vi "ServerMessageParseStateMachine.vi"(0 "LastState":T3, 1 "LastDataBuffer":string, 2 "LastFrameState":T1, 5 "error in":errorcluster) -> (14 "CurrentState":T3, 15 "CurrentDataBuffer":string, 16 "CurrentFrameState":T1, 18 "ReadyFrames":T1[](array[typedef]), 19 "error out":errorcluster)   [LabVIEW 2017, in "STOMP.lvclass"]
uses:
  STOMP.lvclass
  Typedefs/Type_MessageParserState.ctl
  Typedefs/Type_ServerFrame.ctl
  Typedefs/Type_ServerFrameType.ctl
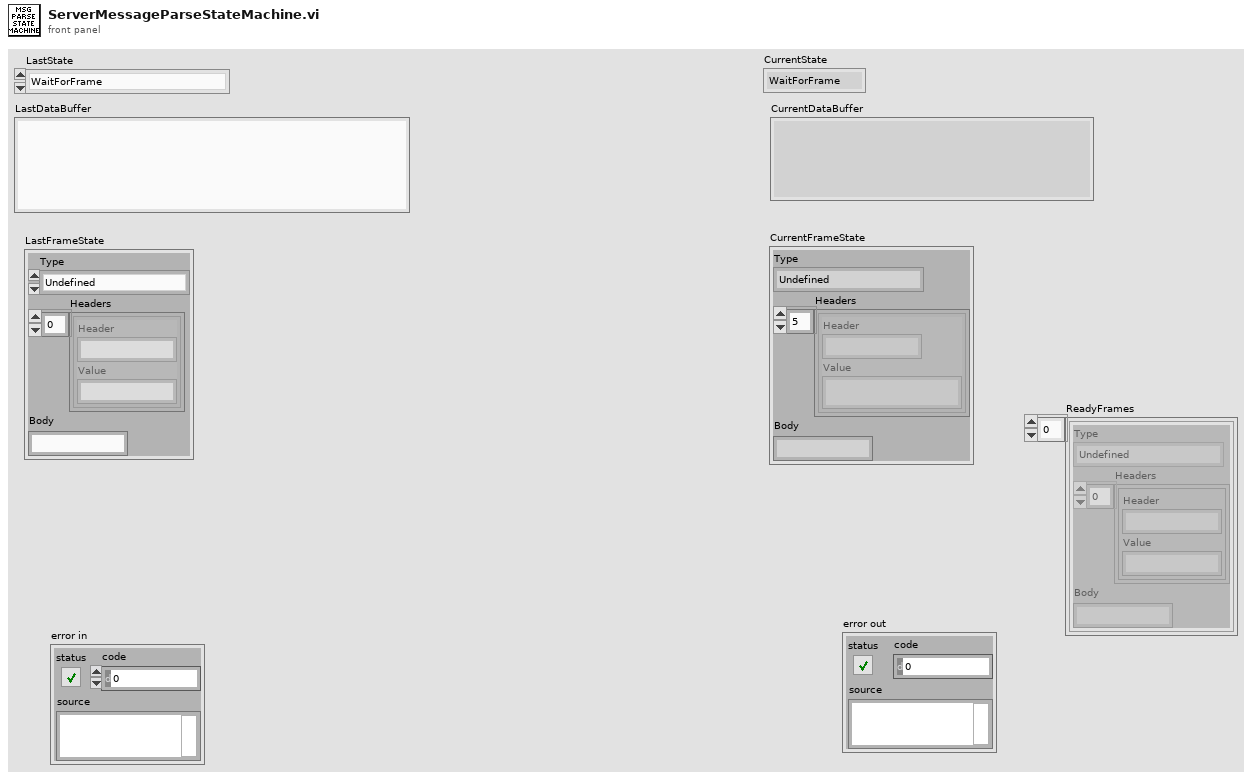
[diagram p1: front panel]
types:
  T1 = typedef "STOMP.lvclass/Type_ServerFrame.ctl" = cluster{"Type":T2, "Headers":cluster{"Header":string, "Value":string}[], "Body":string}
  T2 = typedef "STOMP.lvclass/Type_ServerFrameType.ctl" = enum16{"Undefined", "MESSAGE", "CONNECTED", "RECEIPT", "ERROR"}
  T3 = typedef "STOMP.lvclass/Type_MessageParserState.ctl" = enum16{"WaitForFrame", "ReadCommand", "ReadHeaders", "ReadBody", "FrameReady"}
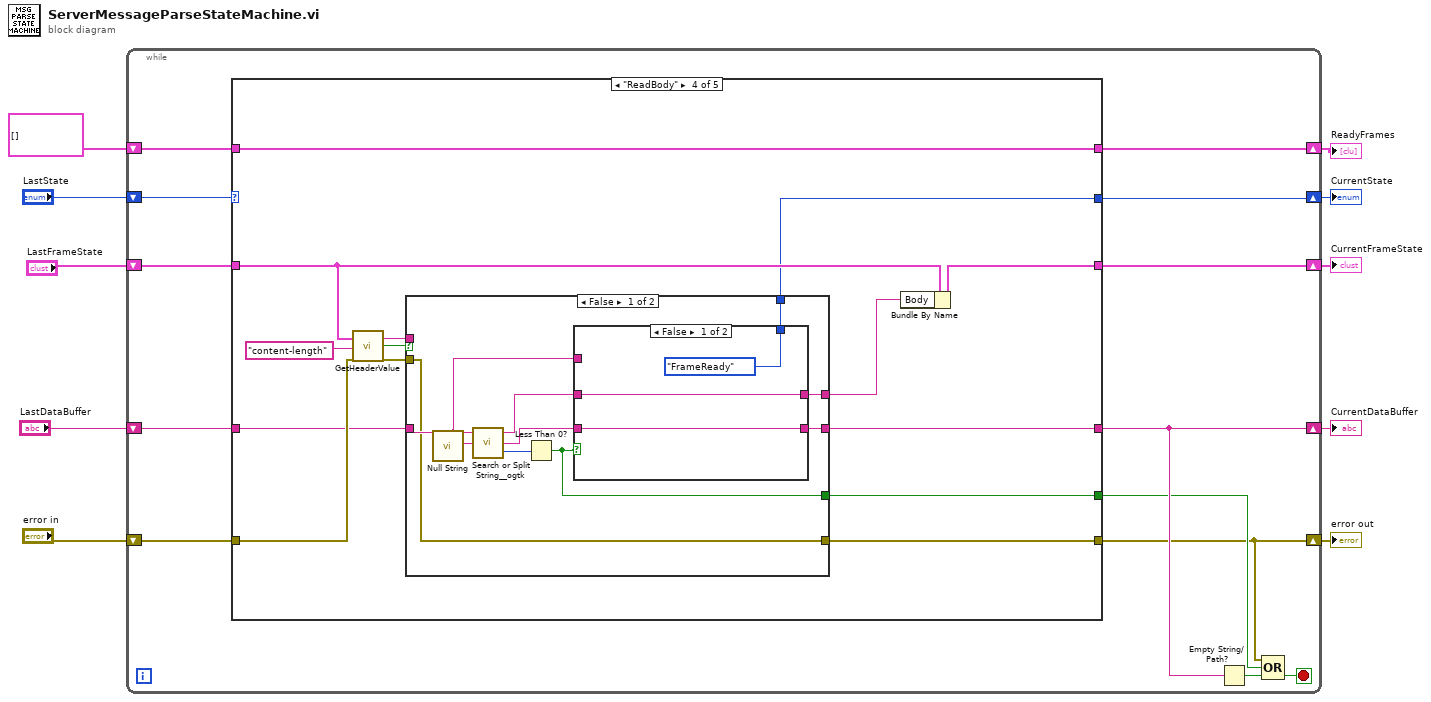
[diagram p0: block diagram]
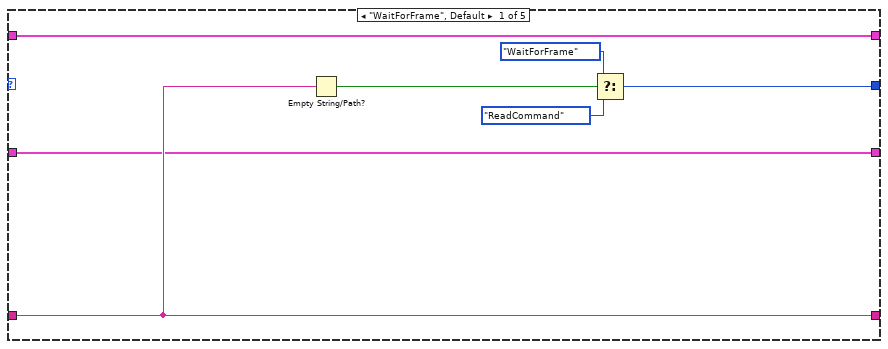
[diagram p2: hidden frame]
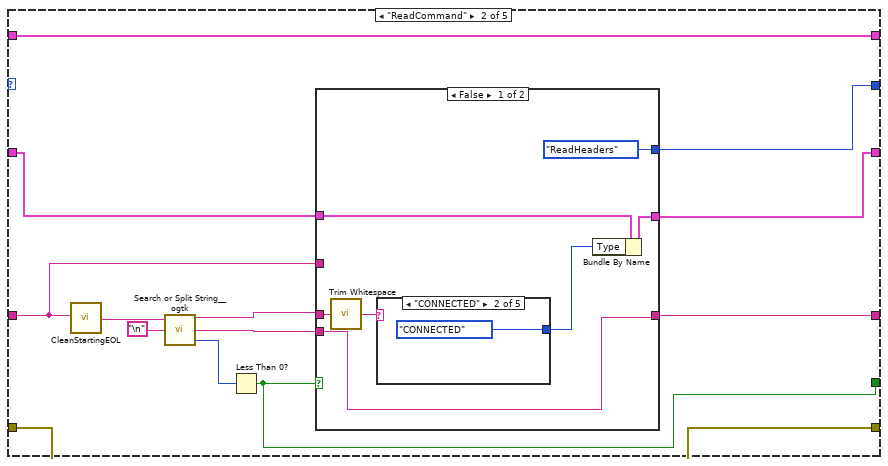
[diagram p3: hidden frame]
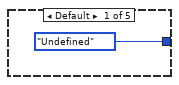
[diagram p4: hidden frame]
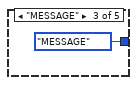
[diagram p5: hidden frame]
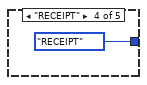
[diagram p6: hidden frame]
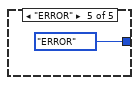
[diagram p7: hidden frame]
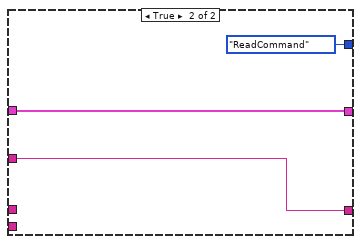
[diagram p8: hidden frame]
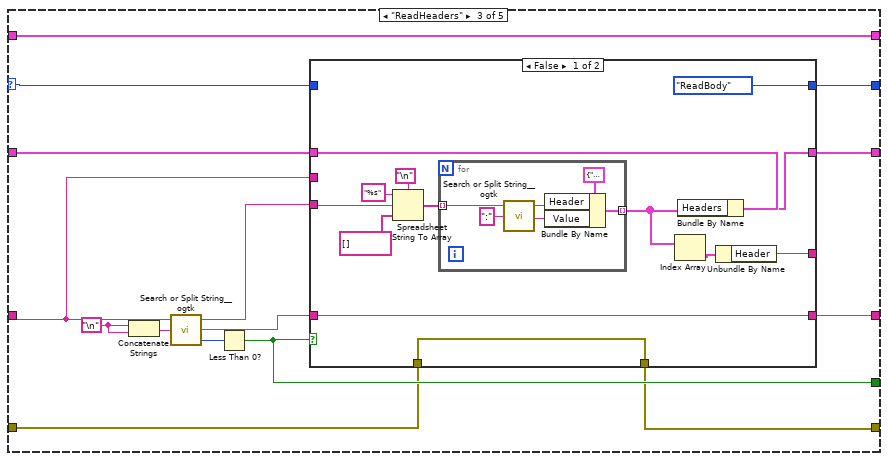
[diagram p9: hidden frame]
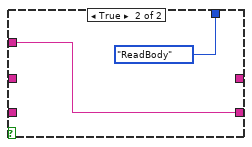
[diagram p11: hidden frame]
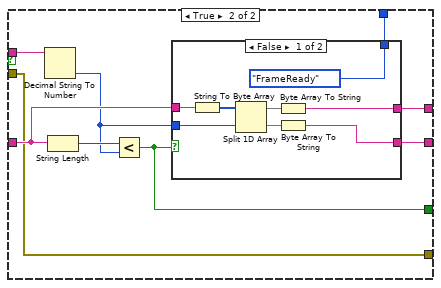
[diagram p12: hidden frame]
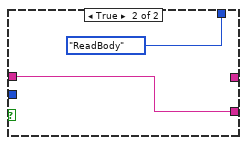
[diagram p13: hidden frame]
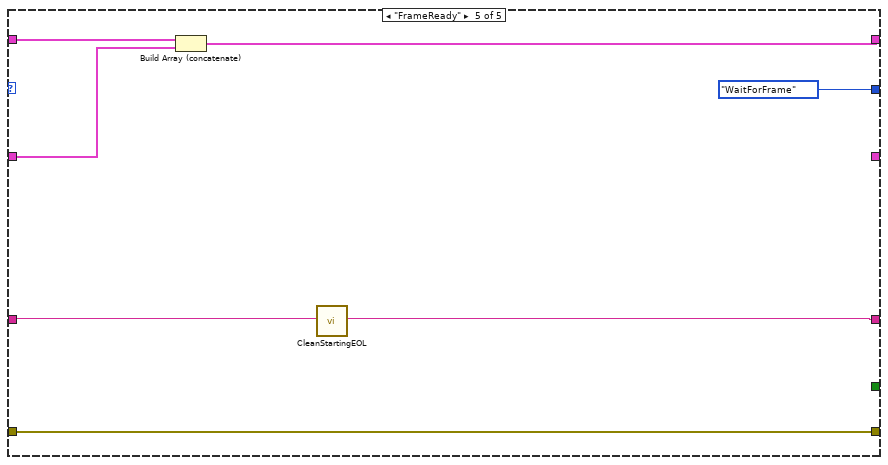
[diagram p14: hidden frame]
diagram:
  n1 = while {
    shift-right: [w21] -> w5
    shift-left: "LastDataBuffer" -> [w22]
    shift-right: [w19] -> w4
    shift-left: "LastState" -> [w23]
    shift-right: [w11] -> w3
    shift-left: "error in" -> [w18]
    shift-right: [w16] -> w6
    shift-left: "LastFrameState" -> [w17]
    shift-right: [w12] -> w1
    shift-left: T1[] [] -> [w13]
    stop <- w15 stop-if-true
    n2 = case shown="\"ReadBody\"" w23 {
      selector: w23 -> [_ _ w64 _ _]
      tunnel: w22 -> [w30 w37 w61 w107 w146]
      tunnel: [w30 w36 w60 w102 w145] -> w21
      tunnel: [w26 w33 w65 w98 Type_MessageParserState."WaitForFrame" ("LastState")] -> w19
      tunnel: w18 -> [_ w31 w62 w109 w147]
      tunnel: w17 -> [w25 w41 w73 w105 w150]
      tunnel: [w25 w40 w72 w104 _] -> w16
      tunnel: [_ w31 w66 w99 w147] -> w11
      tunnel: [_ w34 w68 w101 _] -> w14
      tunnel: w13 -> [w24 w32 w63 w97 w151]
      tunnel: [w24 w32 w63 w97 w149] -> w12
      frame "WaitForFrame", Default {
        n3 = Empty String/Path?(string/path=w30) -> (empty?=w29:bool)
        n4 = Select(t=Type_MessageParserState."WaitForFrame" ("LastState"), s=w29, f=Type_MessageParserState."ReadCommand" ("LastState")) -> (s? t:f=w26:T3)
      }
      frame "ReadCommand" {
        n5 = call "CleanStartingEOL.vi"("String"=w37) -> ("string"=w43:string)  [unwired: 18 in]
        n6 = call <userlib>:"Search or Split String__ogtk.vi"("search string/char (-)"="\n", "string"=w43) -> ("offset after match"=w38:i32, "substring after match"=w35:string, "substring before match"=w39:string)  [unwired: 1 in]
        n7 = Less Than 0?(x=w38) -> (x < 0?=w34:bool)
        n8 = case shown="False" w34 {
          tunnel: w41 -> [w50 w56]
          tunnel: [w49 w56] -> w40
          tunnel: w39 -> [w48 _]
          tunnel: w37 -> [_ w58]
          tunnel: [w45 w58] -> w36
          tunnel: w35 -> [w45 _]
          tunnel: [Type_MessageParserState."ReadHeaders" ("LastState") Type_MessageParserState."ReadCommand" ("LastState")] -> w33
          frame False {
            n9 = call <vilib>:"Trim Whitespace.vi"("string"=w48) -> ("trimmed string"=w47:string)  [unwired: 1 in]
            n10 = case shown="\"CONNECTED\"" w47 {
              tunnel: [Type_ServerFrameType."Undefined" ("Type") Type_ServerFrameType."CONNECTED" ("Type") Type_ServerFrameType."MESSAGE" ("Type") Type_ServerFrameType."RECEIPT" ("Type") Type_ServerFrameType."ERROR" ("Type")] -> w46
              frame Default {
              }
              frame "CONNECTED" {
              }
              frame "MESSAGE" {
              }
              frame "RECEIPT" {
              }
              frame "ERROR" {
              }
            }
            n11 = Bundle By Name(cluster=w50, "Type"=w46) -> (w49:T1)
          }
          frame True {
          }
        }
      }
      frame "ReadHeaders" {
        w69 = "\n"
        n12 = Concatenate Strings(w69, w69) -> (w71:string)
        n13 = call <userlib>:"Search or Split String__ogtk.vi"("search string/char (-)"=w71, "string"=w61) -> ("offset after match"=w70:i32, "substring after match"=w59:string, "substring before match"=w67:string)  [unwired: 1 in]
        n14 = Less Than 0?(x=w70) -> (x < 0?=w68:bool)
        n15 = case shown="False" w68 {
          tunnel: w73 -> [w81 w94]
          tunnel: [w80 w94] -> w72
          tunnel: w67 -> [w86 _]
          tunnel: w62 -> [w78 w96]
          tunnel: [w78 w96] -> w66
          tunnel: [Type_MessageParserState."ReadBody" ("LastState") w95] -> w65
          tunnel: w64 -> [_ w95]
          tunnel: [w75 _] -> _
          tunnel: w61 -> [_ w93]
          tunnel: [w74 w93] -> w60
          tunnel: w59 -> [w74 _]
          frame False {
            n16 = Spreadsheet String To Array(delimiter (Tab)="\n", format string="%s", spreadsheet string=w86, array type (2D Dbl)=string[] []) -> (array=w82:string[])
            n17 = for {
              tunnel: w82 -> [w92] mode=indexing
              tunnel: [w87] -> w77 mode=indexing
              n18 = call <userlib>:"Search or Split String__ogtk.vi"("search string/char (-)"=":" ("regular expression"), "string"=w92) -> ("substring after match"=w88:string, "substring before match"=w89:string)  [unwired: 1 in, 1 out]
              n19 = Bundle By Name(cluster=cluster{"Header":string, "Value":string} {"Header"="", "Value"=""}, "Header"=w89, "Value"=w88) -> (w87:cluster{"Header":string, "Value":string})
            }
            n20 = Index Array(array=w77) -> (element=w76:cluster{"Header":string, "Value":string})  [unwired: 1 in]
            n21 = Bundle By Name(cluster=w81, "Headers"=w77) -> (w80:T1)
            n22 = Unbundle By Name(w76) -> ("Header"=w75:string)
          }
          frame True {
          }
        }
      }
      frame "ReadBody" {
        n23 = call "GetHeaderValue.vi"("Server Frame"=w105, "Header Name"="content-length", "error in"=w109) -> ("Value"=w106:string, "Found?"=w108:bool, "error out"=w100:errorcluster)  [unwired: 14 in]
        n24 = case shown="False" w108 {
          tunnel: w107 -> [w113 w131]
          tunnel: w106 -> [_ w134]
          tunnel: [w116 w129] -> w103
          tunnel: [w114 w128] -> w102
          tunnel: [w118 w132] -> w101
          tunnel: w100 -> [w111 w127]
          tunnel: [w111 w127] -> w99
          tunnel: [w112 w126] -> w98
          frame False {
            n25 = call "Null String.vi"() -> ("NULL"=w120:string)  [unwired: 19 in]
            n26 = call <userlib>:"Search or Split String__ogtk.vi"("search string/char (-)"=w120, "string"=w113) -> ("offset after match"=w119:i32, "substring after match"=w115:string, "substring before match"=w117:string)  [unwired: 1 in]
            n27 = Less Than 0?(x=w119) -> (x < 0?=w118:bool)
            n28 = case shown="False" w118 {
              tunnel: w117 -> [w123 _]
              tunnel: [w123 _] -> w116
              tunnel: w115 -> [w121 _]
              tunnel: [w121 w125] -> w114
              tunnel: w113 -> [_ w125]
              tunnel: [Type_MessageParserState."FrameReady" ("LastState") Type_MessageParserState."ReadBody" ("LastState")] -> w112
              frame False {
              }
              frame True {
              }
            }
          }
          frame True {
            n29 = Decimal String To Number(string=w134) -> (number=w130:i32)  [unwired: 2 in, 1 out]
            n30 = String Length(string=w131) -> (length=w133:i32)
            n31 = Less?(x=w133, y=w130) -> (x < y?=w132:bool)
            n32 = case shown="False" w132 {
              tunnel: w131 -> [w142 w144]
              tunnel: w130 -> [w140 _]
              tunnel: [w138 _] -> w129
              tunnel: [w135 w144] -> w128
              tunnel: [Type_MessageParserState."FrameReady" ("LastState") Type_MessageParserState."ReadBody" ("LastState")] -> w126
              frame False {
                n33 = String To Byte Array(string=w142) -> (unsigned byte array=w141:u8[])
                n34 = Split 1D Array(array=w141, index=w140) -> (first subarray=w139:u8[], second subarray=w137:u8[])
                n35 = Byte Array To String(unsigned byte array=w139) -> (string=w138:string)
                n36 = Byte Array To String(unsigned byte array=w137) -> (string=w135:string)
              }
              frame True {
              }
            }
          }
        }
        n37 = Bundle By Name(cluster=w105, "Body"=w103) -> (w104:T1)
      }
      frame "FrameReady" {
        n38 = Build Array (concatenate)(w151, w150) -> (w149:T1[])
        n39 = call "CleanStartingEOL.vi"("String"=w146) -> ("string"=w145:string)  [unwired: 18 in]
      }
    }
    n40 = Empty String/Path?(string/path=w21) -> (empty?=w20:bool)
    n41 = Compound Arithmetic op=OR(w11, w14, w20) -> (w15:bool)
  }
  "CurrentFrameState" <- w6
  "CurrentDataBuffer" <- w5
  "CurrentState" <- w4
  "error out" <- w3
  "ReadyFrames" <- w1
